vi "Lawofcos.vi"(9 "c":dbl format="%#_13g", 10 "b":dbl format="%#_13g", 11 "a":dbl format="%#_13g") -> (3 "Degrees":dbl)   [LabVIEW 2018]
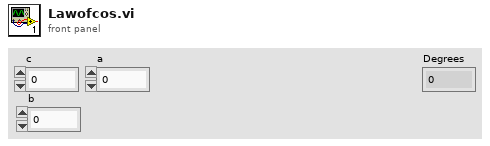
[diagram p1: front panel]
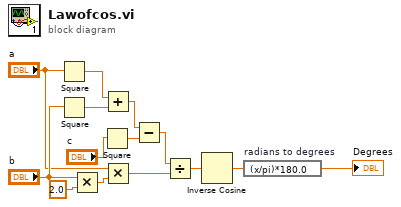
[diagram p0: block diagram]
diagram:
  n1 = Square(x="a") -> (x^2=w13:dbl)
  n2 = Square(x="b") -> (x^2=w12:dbl)
  n3 = Multiply(x="b", y=2.0) -> (x*y=w6:dbl)
  n4 = Square(x="c") -> (x^2=w10:dbl)
  n5 = Add(x=w13, y=w12) -> (x+y=w11:dbl)
  n6 = Multiply(x="a", y=w6) -> (x*y=w4:dbl)
  n7 = Subtract(x=w11, y=w10) -> (x-y=w9:dbl)
  n8 = Divide(x=w9, y=w4) -> (x/y=w3:dbl)
  n9 = Inverse Cosine(1:w3) -> (0:w2:dbl)
  n10 = expression code="(x/pi)*180.0" "radians to degrees"(w2) -> (→"Degrees":dbl)
